vi "Half-Bytes To Byte.vi"(8 "Lower Half-byte":u8 format="%b", 9 "Upper Half-Byte":u8 format="%b") -> (3 "Byte":u8=127 format="%b")   [LabVIEW 2021, in "wamplv.lvlib" / "RawSocket TCP Handler.lvclass"]
uses:
  RawSocket TCP Handler.lvclass
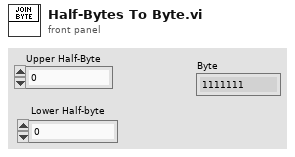
[diagram p1: front panel]
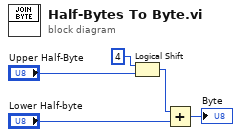
[diagram p0: block diagram]
diagram:
  n1 = Logical Shift(y=i16 4, x="Upper Half-Byte") -> (x << y=w3:u8)
  n2 = Add(x=w3, y="Lower Half-byte") -> (x+y=→"Byte":u8)
